vi "okCFrontPanel Dispose Device Sensors.vi"(8 "Error In":errorcluster, 11 "DeviceSensors Refnum":refnum<k24>) -> (0 "Error Out":errorcluster)   [LabVIEW 2021, in "okFrontPanelC#Wrapper.lvlib"]
uses:
  okFrontPanelC#Wrapper.lvlib
  D:/UCLA Thinkpad Google Drive/LabVIEW 2021 SP1/builds/SwissSPAD Live Distribution/Opal Kelly/C# Wrapper/v5.0.2/libFrontPanel-csharp.dll
  v5.0.2/libFrontPanel-csharp.dll
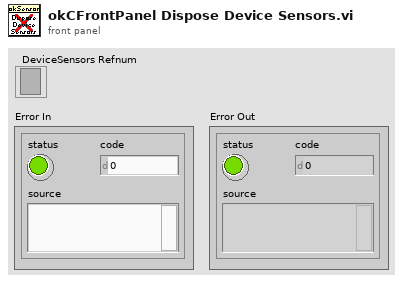
[diagram p1: front panel]
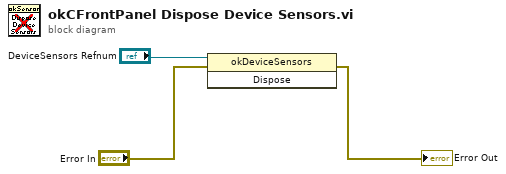
[diagram p0: block diagram]
diagram:
  n1 = invoke class="okDeviceSensors" method="Dispose"(reference="DeviceSensors Refnum", error in="Error In") -> (error out=→"Error Out":errorcluster)  [unwired: 1 in, 2 out]
